vi "VCO_Test.vi"() -> ()   [LabVIEW 2012]
panel:
  out "Freq":dbl
  out "VCO Frequency Chart 2":dbl(graph)
  out "Sinz Chart":ext(graph)
  out "true f":dbl
  out "z":dbl
  out "cos(z)":dbl
  in  "VCO nominal freq":dbl
  out "nominal freq. indicator":dbl
  in  "Sampling Frequency":dbl
  in  "Nominal Frequency":dbl
  in  "Alpha":dbl
  in  "PID Error":dbl
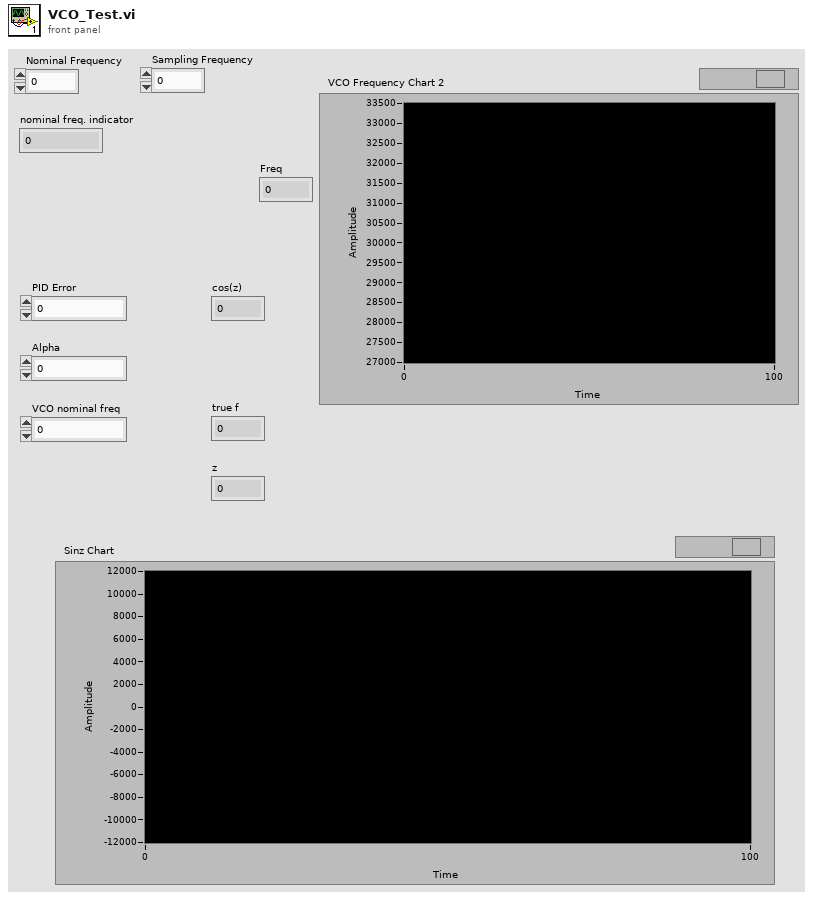
[diagram p1: front panel]
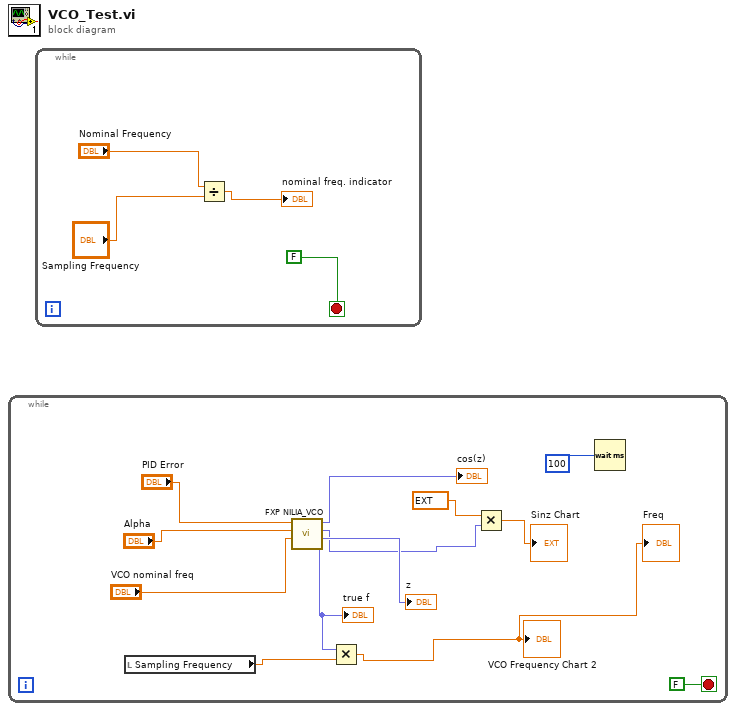
[diagram p0: block diagram]
diagram:
  n1 = while {
    stop <- FALSE stop-if-true
    n2 = local read "Sampling Frequency"() -> (w6:dbl)
    n3 = call "FXP NILIA_VCO.vi"("nominal freq [U16.0]"="VCO nominal freq", "Kv [U16.0]"="Alpha", "v [I32.17]"="PID Error") -> ("f"=w7:fxp<+/-,32,0>, "z [I32.1]"=→"z":fxp<+/-,32,1>, "sin(z) [I16.2]"=w2:fxp<+/-,16,2>, "cos(z) [I16.2]"=→"cos(z)":fxp<+/-,16,2>)  [unwired: 5 in]
    "true f" <- w7
    n4 = Multiply(x=w7, y=w6) -> (x*y=→"VCO Frequency Chart 2" →"Freq":dbl)
    n5 = Multiply(x=ext 10814.0, y=w2) -> (x*y=→"Sinz Chart":ext)
    n6 = Wait (ms)(milliseconds to wait=100) -> ()  [unwired: 1 out]
  }
  n7 = while {
    stop <- FALSE ("Nominal Frequency") stop-if-true
    n8 = Divide(x="Nominal Frequency", y="Sampling Frequency") -> (x/y=→"nominal freq. indicator":dbl)
  }
